vi "Construct.vi"(6 "Labels":map{string, string}(c390), 8 "error in (no error)":errorcluster, 9 "Timestamp":timestamp format="%<%x %.3X>T", 10 "Value":dbl, 11 "Name":string) -> (0 "error out":errorcluster, 3 "Sample out":refnum<class "Sample.lvclass">)   [LabVIEW 2020, in "Metrics.lvlib" / "Sample.lvclass"]
uses:
  Sample.lvclass
  Sample.lvclass/Sample.ctl
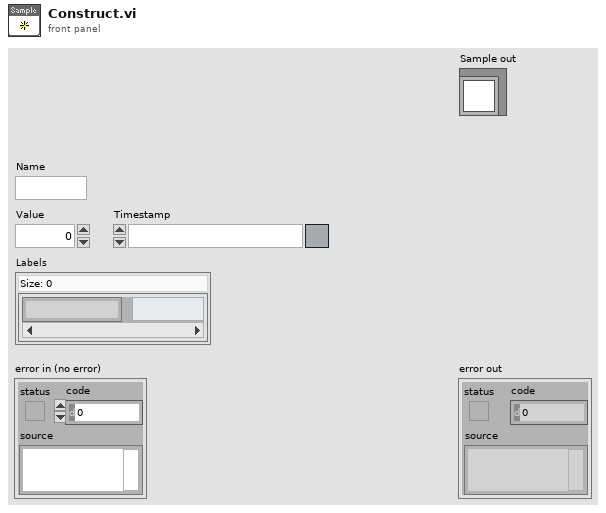
[diagram p1: front panel]
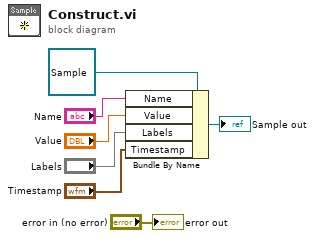
[diagram p0: block diagram]
diagram:
  n1 = Bundle By Name(cluster=refnum<class "Sample.lvclass"> refnum ("Sample in"), "Name"="Name", "Value"="Value", "Labels"="Labels", "Timestamp"="Timestamp") -> (→"Sample out":refnum<class "Sample.lvclass">)
  "error out" <- "error in (no error)"
